vi "Update obsticles.vi"(6 "angle input":dbl, 8 "Robot Location":dbl[](array[numeric]), 9 "p":dbl, 10 "Map Input":dbl[][](array[numeric]), 11 "Object location":dbl[][](array[numeric])) -> (3 "Map output":dbl[][](array[numeric]))   [LabVIEW 2015]
panel:
  out "length":dbl
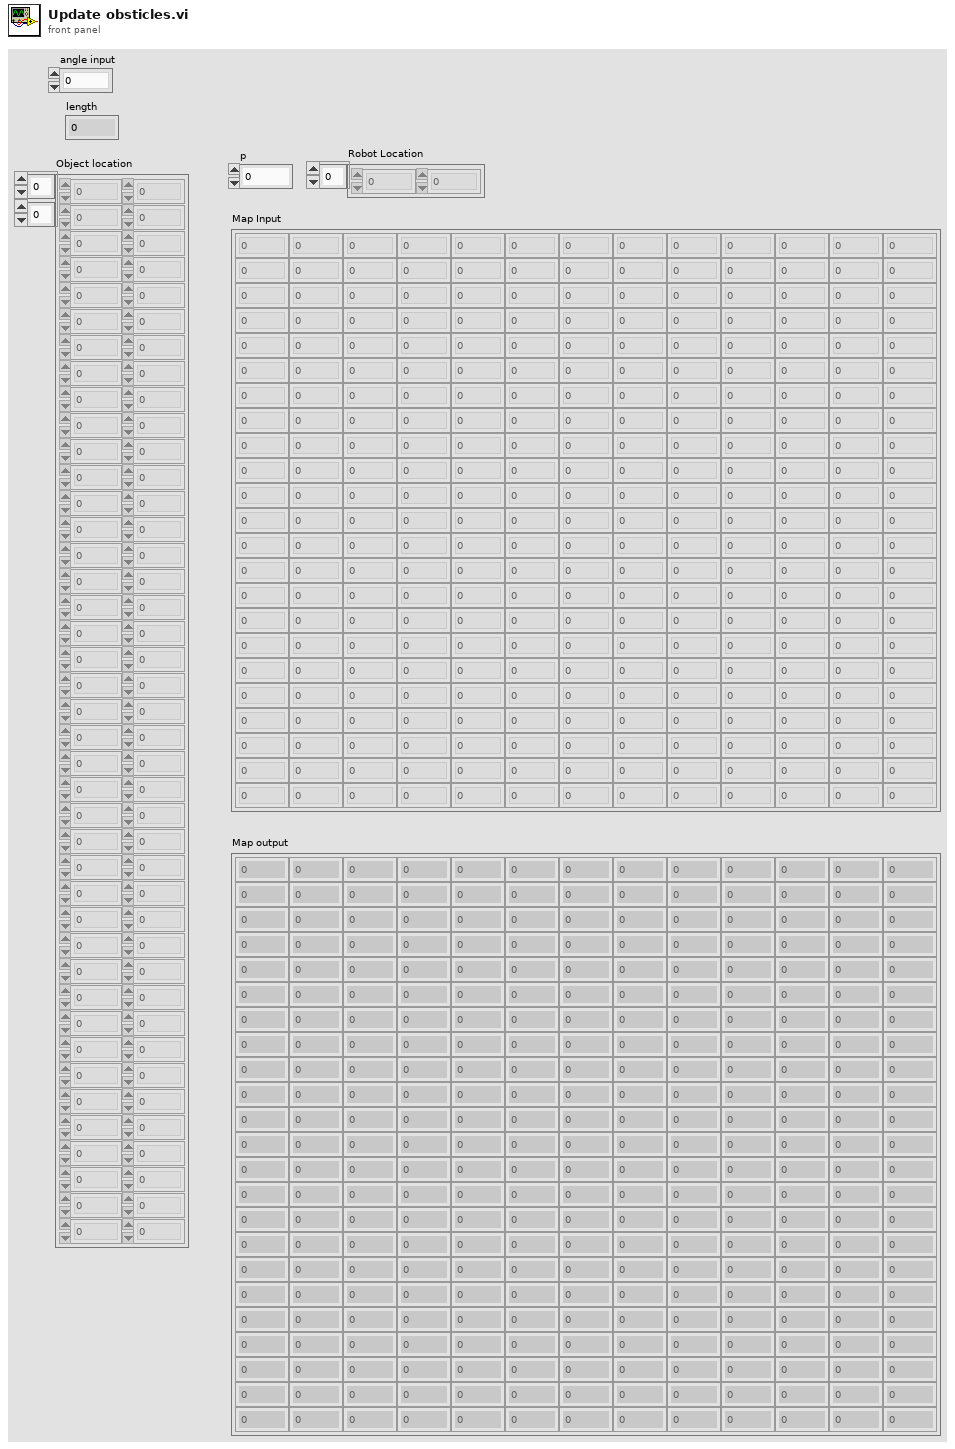
[diagram p1: front panel]
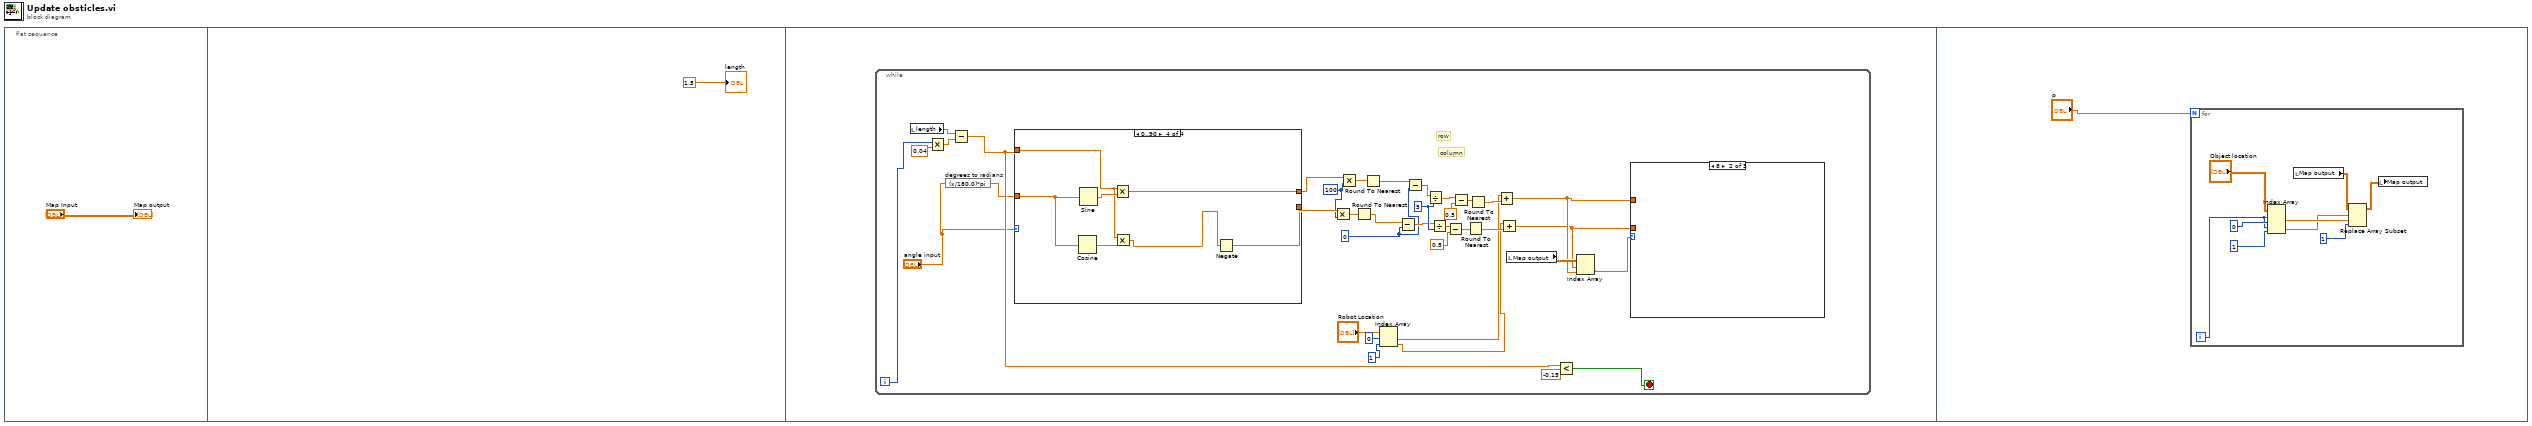
[diagram p0: block diagram]
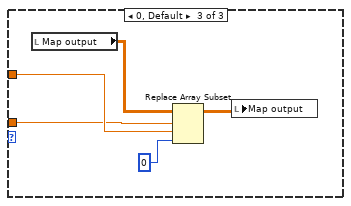
[diagram p3: hidden frame]
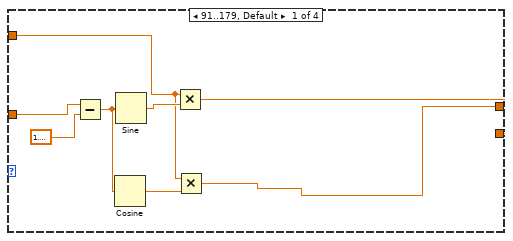
[diagram p4: hidden frame]
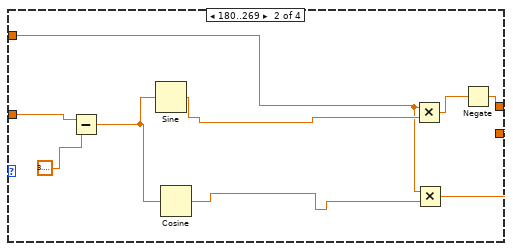
[diagram p5: hidden frame]
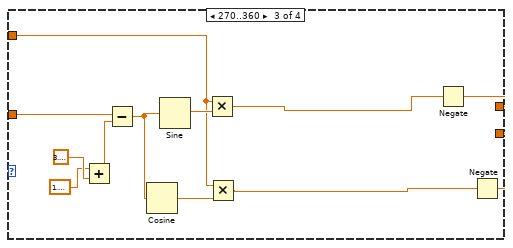
[diagram p6: hidden frame]
diagram:
  n1 = flat-sequence {
    frame #0 {
      "Map output" <- "Map Input"
    }
    frame #1 {
      "length" <- 1.5
    }
    frame #2 {
      n2 = while {
        i -> [w13]
        stop <- w10 stop-if-true
        w21 = 0
        w37 = 100
        w39 = 5
        # "column"
        # "row"
        n3 = local read "length"() -> (w15:dbl)
        n4 = Multiply(x=w13, y=0.04) -> (x*y=w14:dbl)
        n5 = expression code="(x/180.0)*pi" "degrees to radians"("angle input") -> (w3:dbl)
        n6 = Subtract(x=w15, y=w14) -> (x-y=w12:dbl)
        n7 = case shown="0..90" "angle input" {
          tunnel: w3 -> [w49 w60 w69 w79]
          tunnel: w12 -> [w45 w53 w61 w73]
          tunnel: [w46 w58 w62 w77] -> w20
          tunnel: [w47 w57 w63 w75] -> w38
          frame 91..179, Default {
            n8 = Subtract(x=w49, y=1.5707963267948966) -> (x-y=w50:dbl)
            n9 = Cosine(x=w50) -> (cos(x)=w51:dbl)
            n10 = Sine(x=w50) -> (sin(x)=w52:dbl)
            n11 = Multiply(x=w45, y=w52) -> (x*y=w47:dbl)
            n12 = Multiply(x=w45, y=w51) -> (x*y=w46:dbl)
          }
          frame 180..269 {
            n13 = Subtract(x=w60, y=3.141592653589793) -> (x-y=w56:dbl)
            n14 = Sine(x=w56) -> ()  [unwired: 1 out]
            n15 = Cosine(x=w56) -> (cos(x)=w55:dbl)
            n16 = Multiply(x=w53, y=w56) -> (x*y=w59:dbl)
            n17 = Multiply(x=w53, y=w55) -> (x*y=w57:dbl)
            n18 = Negate(x=w59) -> (-x=w58:dbl)
          }
          frame 270..360 {
            n19 = Add(x=1.5707963267948966, y=3.141592653589793) -> (x+y=w64:dbl)
            n20 = Subtract(x=w69, y=w64) -> (x-y=w72:dbl)
            n21 = Cosine(x=w72) -> (cos(x)=w71:dbl)
            n22 = Sine(x=w72) -> (sin(x)=w70:dbl)
            n23 = Multiply(x=w61, y=w70) -> (x*y=w67:dbl)
            n24 = Multiply(x=w61, y=w71) -> (x*y=w68:dbl)
            n25 = Negate(x=w67) -> (-x=w63:dbl)
            n26 = Negate(x=w68) -> (-x=w62:dbl)
          }
          frame 0..90 {
            n27 = Cosine(x=w79) -> (cos(x)=w74:dbl)
            n28 = Sine(x=w79) -> (sin(x)=w78:dbl)
            n29 = Multiply(x=w73, y=w78) -> (x*y=w77:dbl)
            n30 = Multiply(x=w73, y=w74) -> (x*y=w76:dbl)
            n31 = Negate(x=w76) -> (-x=w75:dbl)
          }
        }
        n32 = Multiply(x=w38, y=w37) -> (x*y=w17:dbl)
        n33 = Multiply(x=w20, y=w37) -> (x*y=w19:dbl)
        n34 = Round To Nearest(number=w17) -> (nearest integer value=w16:dbl)
        n35 = Round To Nearest(number=w19) -> (nearest integer value=w18:dbl)
        n36 = Index Array(array="Robot Location", index #1=0, index #2=1) -> (element #1=w25:dbl, element #2=w24:dbl)
        n37 = Subtract(x=w16, y=w21) -> (x-y=w22:dbl)
        n38 = Subtract(x=w18, y=w21) -> (x-y=w23:dbl)
        n39 = Divide(x=w23, y=w39) -> (x/y=w30:dbl)
        n40 = Divide(x=w22, y=w39) -> (x/y=w34:dbl)
        n41 = Subtract(x=w34, y=0.5) -> (x-y=w33:dbl)
        n42 = Subtract(x=w30, y=0.5) -> (x-y=w29:dbl)
        n43 = Round To Nearest(number=w33) -> (nearest integer value=w36:dbl)
        n44 = Round To Nearest(number=w29) -> (nearest integer value=w35:dbl)
        n45 = Add(x=w25, y=w35) -> (x+y=w8:dbl)
        n46 = Add(x=w24, y=w36) -> (x+y=w7:dbl)
        n47 = local read "Map output"() -> (w9:dbl[][])
        n48 = Less?(x=w12, y=-0.15) -> (x < y?=w10:bool)
        n49 = Index Array(array=w9, index (row)=w7, index (col)=w8) -> (element=w5:dbl)
        n50 = case shown="8" w5 {
          tunnel: w8 -> [_ _ w41]
          tunnel: w7 -> [_ _ w40]
          frame 1 {
          }
          frame 8 {
          }
          frame 0, Default {
            n51 = local read "Map output"() -> (w44:dbl[][])
            n52 = Replace Array Subset(array=w44, new element=0, index (row)=w40, index (col)=w41) -> (w43:dbl[][])
            n53 = local write "Map output"(w43) -> ()
          }
        }
      }
    }
    frame #3 {
      n54 = for {
        N: "p" -> [_]
        i -> [w84]
        n55 = Index Array(array="Object location", index (row) #1=w84, index (col) #1=0, index (row) #2=w84, index (col) #2=1) -> (element #1=w83:dbl, element #2=w82:dbl)
        n56 = local read "Map output"() -> (w89:dbl[][])
        n57 = Replace Array Subset(array=w89, new element=1, index (row)=w82, index (col)=w83) -> (w88:dbl[][])
        n58 = local write "Map output"(w88) -> ()
      }
    }
  }
